vi "Call Serial Decoder Read Only.vi"(0 "VISA resource name":refnum<visa-resource-name>, 1 "milliseconds to wait":u32=500, 3 "error in":errorcluster={"status"=FALSE, "code"=-1073807343, "source"=""}) -> (5 "Data Read":T1={"Date"="03/29/13", "Time"="14:47:22", "CO2- ppm"=753, "Last Ctrl Word"=5276928, "O2-1 ppm"=209104, "O2-2 ppm"=209104, "Temp MB"=20.41, "Temp Sensor Modulr"=21.85, "Press mB"=835.52} {"Last Ctrl Word" format="%.0x"}, 6 "VISA resource name out":refnum<visa-resource-name>, 7 "error out":errorcluster={"status"=FALSE, "code"=-1073807343, "source"=""})   [LabVIEW 2012]
panel:
  out "read buffer":string="03/29/13,14:47:22,753, 00508500, 209104, 209104, 20.41, 21.85, 835.52\r\n"
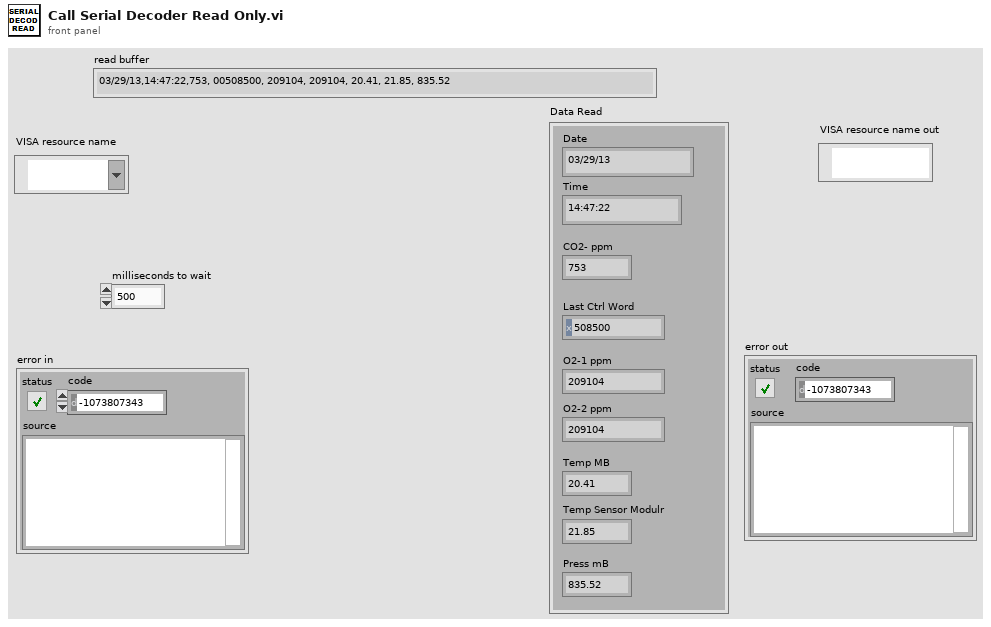
[diagram p1: front panel]
types:
  T1 = cluster{"Date":string, "Time":string, "CO2- ppm":u32, "Last Ctrl Word":u32, "O2-1 ppm":u32, "O2-2 ppm":u32, "Temp MB":sgl, "Temp Sensor Modulr":sgl, "Press mB":sgl}
  T2 = cluster{"default value 1":string, "default value 1":string, "default value 5":u32, "default value 5":u32, "default value 5":u32, "default value 5":u32, "default value 7":sgl, "default value 7":sgl, "default value 7":sgl}
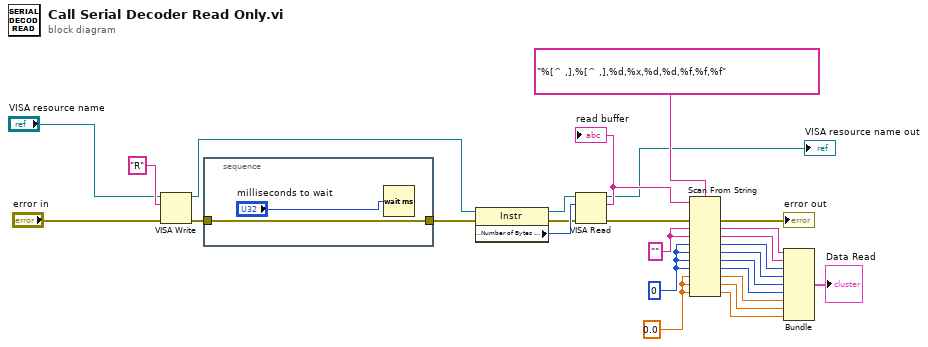
[diagram p0: block diagram]
diagram:
  w7 = sgl 0.0 ("default value 7")
  w20 = "" ("default value 1")
  w6 = u32 0 ("default value 5")
  n1 = VISA Write(VISA resource name="VISA resource name", write buffer="R" ("string"), error in (no error)="error in") -> (VISA resource name out=w18:refnum<visa-resource-name>, error out=w19:errorcluster)  [unwired: 1 out]
  n2 = stacked-sequence {
    tunnel: [w28] -> w21
    tunnel: w19 -> [w28]
    frame #0 {
      n3 = Wait (ms)(milliseconds to wait="milliseconds to wait") -> ()  [unwired: 1 out]
    }
  }
  n4 = property class="Instr"(reference=w18, error in=w21) -> (reference out=w23:refnum<visa-resource-name>, error out=w22:errorcluster, "Serial Settings:Number of Bytes at Serial Port"=w24:u32)
  n5 = VISA Read(VISA resource name=w23, byte count=w24, error in (no error)=w22) -> (VISA resource name out=→"VISA resource name out":refnum<visa-resource-name>, read buffer=w26:string, error out=w2:errorcluster)  [unwired: 1 out]
  "read buffer" <- w26
  n6 = Scan From String(format string="%[^ ,],%[^ ,],%d,%x,%d,%d,%f,%f,%f" ("String"), input string=w26, error in=w2, default 1=w20, default 2=w20, default 3=w6, default 4=w6, default 5=w6, default 6=w6, default 7=w7, default 8=w7, default 9=w7) -> (error out=→"error out":errorcluster, output 1=w17:string, output 2=w16:string, output 3=w15:u32, output 4=w14:u32, output 5=w13:u32, output 6=w12:u32, output 7=w11:sgl, output 8=w10:sgl, output 9=w9:sgl)  [unwired: 1 in, 2 out]
  n7 = Bundle("default value 1"=w17, "default value 1"=w16, "default value 5"=w15, "default value 5"=w14, "default value 5"=w13, "default value 5"=w12, "default value 7"=w11, "default value 7"=w10, "default value 7"=w9) -> (→"Data Read":T2)  [unwired: 1 in]
